vi "clear.vi"(8 "error in (no error)":errorcluster, 11 "Bucket in":refnum<class "Bucket.lvclass">) -> (0 "error out":errorcluster, 3 "Bucket out":refnum<class "Bucket.lvclass">)   [LabVIEW 2017, in "Bucket.lvclass"]
uses:
  <userlib>/836-Library/Data_Structures/HashMap/Support/Bucket/Bucket.lvclass
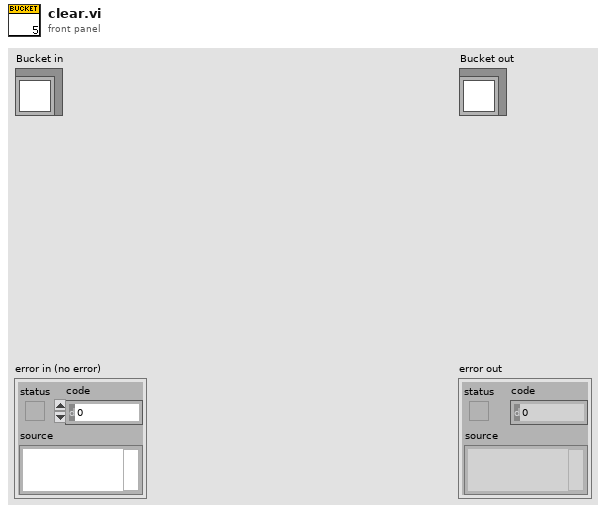
[diagram p1: front panel]
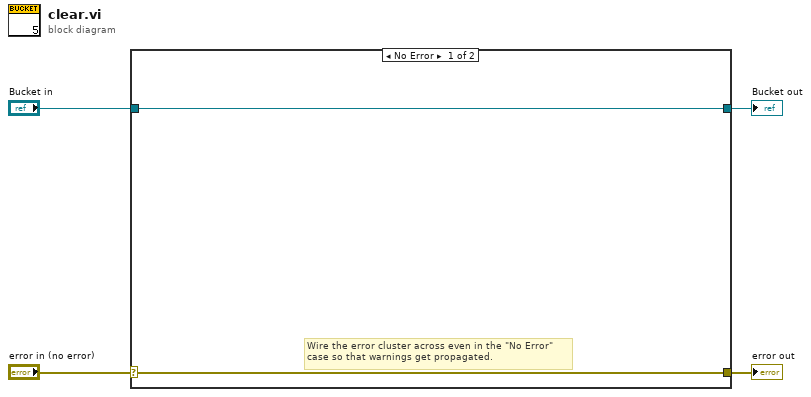
[diagram p0: block diagram]
diagram:
  n1 = case shown="No Error" "error in (no error)" {
    selector: "error in (no error)" -> [w5 w8]
    tunnel: [w5 w8] -> w3
    tunnel: [w6 w7] -> w1
    tunnel: "Bucket in" -> [w6 w7]
    frame No Error {
      # "Wire the error cluster across even in the \"No Error\"\ncase so that warnings get propagated."
    }
    frame Error {
    }
  }
  "error out" <- w3
  "Bucket out" <- w1
